vi "Read GPIO Input Pin.vi"(8 "error in (no error)":errorcluster, 11 "VISA resource name":refnum<visa-resource-name>) -> (0 "error out":errorcluster, 2 "GPIO Input Pin":bool[](array[boolean]), 3 "VISA resource name out":refnum<visa-resource-name>)   [LabVIEW 2013, in "Ocean Optics 2000 4000.lvlib"]
doc: "Returns the status of the GPIO Input Pins"
uses:
  <instrlib>/Ocean Optics 2000 4000/Ocean Optics 2000 4000.lvlib
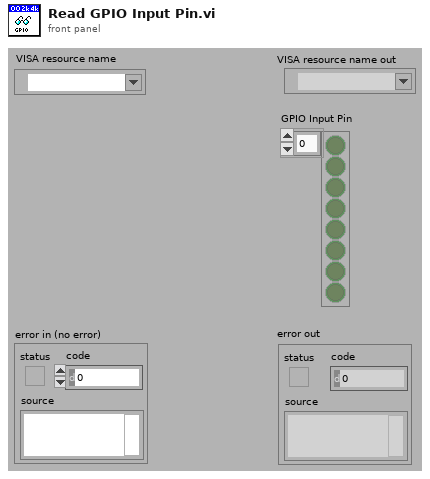
[diagram p1: front panel]
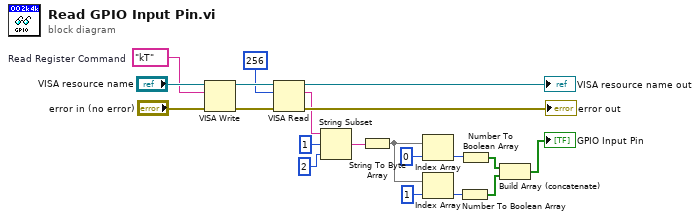
[diagram p0: block diagram]
diagram:
  w19 = "kT"  # Read Register Command
  n1 = VISA Write(VISA resource name="VISA resource name", write buffer=w19, error in (no error)="error in (no error)") -> (VISA resource name out=w17:refnum<visa-resource-name>, error out=w15:errorcluster)  [unwired: 1 out]
  n2 = VISA Read(VISA resource name=w17, byte count=u32 256, error in (no error)=w15) -> (VISA resource name out=→"VISA resource name out":refnum<visa-resource-name>, read buffer=w12:string, error out=→"error out":errorcluster)  [unwired: 1 out]
  n3 = String Subset(string=w12, offset (0)=1, length (rest)=2 ("length (rest)")) -> (substring=w9:string)
  n4 = String To Byte Array(string=w9) -> (unsigned byte array=w7:u8[])
  n5 = Index Array(array=w7, index=0) -> (element=w5:u8)
  n6 = Index Array(array=w7, index=1) -> (element=w4:u8)
  n7 = Number To Boolean Array(number=w4) -> (Boolean array=w2:bool[])
  n8 = Number To Boolean Array(number=w5) -> (Boolean array=w3:bool[])
  n9 = Build Array (concatenate)(w3, w2) -> (→"GPIO Input Pin":bool[])
